vi "Configure Signal (Common).vi"(0 "niUsrpRio Session":T3={"FPGA Interface"=refnum, "RIO Interface Number"=0, "Data Clock Rate"=0, "FPGA Data Clock Rate"=0, "Global Settings Register Bus"=refnum, "Radio 0 Settings Register Bus"=refnum, "Radio 1 Settings Register Bus"=refnum, "Radio Settings Bus Semaphore"=refnum, "DB Queues"=[], "Characterization Data Valid?"=FALSE, "EEPROM Header"={"Checksum"=0, "Product Code"=0, "Hardware Current Version"=0, "Hardware Oldest Compatible Version"=0, "EEPROM Map Current Version"=0, "EEPROM Map Oldest Compatible Version"=0, "User Password"="", "Pointer to Factory Header"=0, "Pointer to User Header"=0, "Recommended Interval"=0, "Number of Reserved Bytes"=9, "Number of Daughterboards"=0, "Daughterboard IDs"=[], "Daughterboard Serial Numbers"=[]}, "Device Data Header"={"Checksum"=0, "Number of Channels"=0, "Number of Gain Settings"=[], "Pointer to Characterization Data"=[], "Number of Reserved Bytes"=27, "Number of Frequencies"=[]}, "EEPROM Characterization Header"={"Checksum"=0, "Date"=timestamp(0 s since 1904-01-01), "Temperature"=0.0, "Misc. Info"="", "Pointer to Device Data Header"=0, "Number of Reserved Bytes"=28}, "Characterization Data"=[], "FPGA Current Version"=0, "FPGA Oldest Compatible Version"=0, "Fixed Logic Current Version"=0, "Fixed Logic Oldest Compatible Version"=0, "FPGA Radio Settings Bus Current Version"=0, "FPGA Radio Settings Bus Oldest Compatible Version"=0, "FPGA Board Config Current Version"=0, "FPGA Board Config Oldest Compatible Version"=0, "Daughterboard Clock Rate"=0, "daughterboard configuration session handles"=[]} {"Daughterboard Clock Rate" format="%#.3pHz"; "FPGA Data Clock Rate" format="%#.3pHz"; "Data Clock Rate" format="%#.3pHz"; "Characterization Data"."Frequencies [Hz]" format="%#_6p"; "EEPROM Characterization Header"."Pointer to Device Data Header" format="%x"; "EEPROM Characterization Header"."Checksum" format="%x"; "Device Data Header"."Pointer to Characterization Data" format="%x"; "Device Data Header"."Checksum" format="%x"; "EEPROM Header"."Pointer to User Header" format="%x"; "EEPROM Header"."Pointer to Factory Header" format="%x"; "EEPROM Header"."Product Code" format="%x"; "EEPROM Header"."Checksum" format="%x"}, 1 "scope":string(combo)="rx", 2 "Correct Impairments?":bool=TRUE, 5 "signal parameters":T2={"gain/level"=0.0, "sample rate [S/s]"=10000000.0, "frequency [Hz]"=2450000000.0, "LO frequency [Hz]"=-1.0, "active antenna"="RX1"} {"LO frequency [Hz]" format="%#.3pHz"; "frequency [Hz]" format="%#.3pHz"; "sample rate [S/s]" min=1.0 max=250000000.0 format="%#.3pS/s"}, 7 "Configure Signal Mode":T1, 11 "error in":errorcluster) -> (4 "niUsrpRio Session (out)":T3={"FPGA Interface"=refnum, "RIO Interface Number"=0, "Data Clock Rate"=0, "FPGA Data Clock Rate"=0, "Global Settings Register Bus"=refnum, "Radio 0 Settings Register Bus"=refnum, "Radio 1 Settings Register Bus"=refnum, "Radio Settings Bus Semaphore"=refnum, "DB Queues"=[], "Characterization Data Valid?"=FALSE, "EEPROM Header"={"Checksum"=0, "Product Code"=0, "Hardware Current Version"=0, "Hardware Oldest Compatible Version"=0, "EEPROM Map Current Version"=0, "EEPROM Map Oldest Compatible Version"=0, "User Password"="", "Pointer to Factory Header"=0, "Pointer to User Header"=0, "Recommended Interval"=0, "Number of Reserved Bytes"=9, "Number of Daughterboards"=0, "Daughterboard IDs"=[], "Daughterboard Serial Numbers"=[]}, "Device Data Header"={"Checksum"=0, "Number of Channels"=0, "Number of Gain Settings"=[], "Pointer to Characterization Data"=[], "Number of Reserved Bytes"=27, "Number of Frequencies"=[]}, "EEPROM Characterization Header"={"Checksum"=0, "Date"=timestamp(0 s since 1904-01-01), "Temperature"=0.0, "Misc. Info"="", "Pointer to Device Data Header"=0, "Number of Reserved Bytes"=28}, "Characterization Data"=[], "FPGA Current Version"=0, "FPGA Oldest Compatible Version"=0, "Fixed Logic Current Version"=0, "Fixed Logic Oldest Compatible Version"=0, "FPGA Radio Settings Bus Current Version"=0, "FPGA Radio Settings Bus Oldest Compatible Version"=0, "FPGA Board Config Current Version"=0, "FPGA Board Config Oldest Compatible Version"=0, "Daughterboard Clock Rate"=0, "daughterboard configuration session handles"=[]} {"Daughterboard Clock Rate" format="%#.3pHz"; "FPGA Data Clock Rate" format="%#.3pHz"; "Data Clock Rate" format="%#.3pHz"; "Characterization Data"."Frequencies [Hz]" format="%#_6p"; "EEPROM Characterization Header"."Pointer to Device Data Header" format="%x"; "EEPROM Characterization Header"."Checksum" format="%x"; "Device Data Header"."Pointer to Characterization Data" format="%x"; "Device Data Header"."Checksum" format="%x"; "EEPROM Header"."Pointer to User Header" format="%x"; "EEPROM Header"."Pointer to Factory Header" format="%x"; "EEPROM Header"."Product Code" format="%x"; "EEPROM Header"."Checksum" format="%x"}, 6 "coerced signal parameters":T2={"gain/level"=0.0, "sample rate [S/s]"=10000000.0, "frequency [Hz]"=2450000000.0, "LO frequency [Hz]"=-1.0, "active antenna"="RX1"} {"LO frequency [Hz]" format="%#.3pHz"; "frequency [Hz]" format="%#.3pHz"; "sample rate [S/s]" min=1.0 max=250000000.0 format="%#.3pS/s"}, 15 "error out":errorcluster)   [LabVIEW 2021]
doc: "Configures the DSP and signal path for the channel based on the input <B>signal parameters</B>.\n\n<B>Input Parameters</B>\n\n<B>Sample Rate</B> the requested rate, in samples per second, the signal will be sampled at.\n\n<B>Frequency</B> is the requested frequency, in hertz, to acquire the signal from/generate the signal at.\n\n<B>Level</B> is the requested power level, in dBm, of the signal.\n\n<B>Gain</B> is the requested amount of gain, in dB.\n\n<B>LO Frequency</B> is the requested frequency, in hertz, to tune the local oscillator to. The default value of -1 sets the LO to the value of the 'Frequency' input. If the value is not -1, the LO will be set to that value, and the DSP will handle the difference between the 'Frequency' and the 'LO Frequency'.\n\n<B>Active Antenna</B> is the antenna to use for this channel.\n\n<B>Correct Impairments</B> applies the correction information of the device to the signal."
uses:
  <instrlib>/niUsrpRio/Config/v1/Host/Public/niUsrpRio Session.ctl
  <instrlib>/_niInstr/Register Bus/v0/Host/Public/Register Bus Session.ctl
  <instrlib>/_niInstr/Register Bus/v0/Host/Private/Session Data.ctl
  <instrlib>/niUsrpRio/Config/v1/Host/Private/DB Queue Reference.ctl
  <instrlib>/niUsrpRio/Config/v1/Host/Private/Daughterboard Data.ctl
  <instrlib>/niUsrpRio/Config/v1/Host/Private/ATR state data.ctl
  <instrlib>/niUsrpRio/Config/v1/Host/Private/Antenna Configuration.ctl
  <instrlib>/niUsrpRio/Config/v1/Host/Private/CPLD Power Mode.ctl
  <instrlib>/niUsrpRio/Config/v1/Host/Public/EEPROM Header.ctl
  <instrlib>/niUsrpRio/Config/v1/Host/Public/EEPROM Device Data Header.ctl
  <instrlib>/niUsrpRio/Config/v1/Host/Public/EEPROM Characterization Header.ctl
  <instrlib>/niUsrpRio/Config/v1/Host/Public/Characterization Data.ctl
  <instrlib>/niUsrpRio/Config/v1/Host/Public/IQ Imbalance.ctl
  Configure Signal Parameters.ctl
  Configure Signal Mode.ctl
  Streaming Xvcr FPGA Ref.ctl
  <instrlib>/_niInstr/DSP/v1/Shared/Public/IQ Impairments.ctl
  <instrlib>/_niInstr/DSP/v1/Shared/Public/IQ Gain.ctl
  <vilib>/Utility/error.llb/Error Cluster From Error Code.vi
  <vilib>/rvi/errors/niLvFpgaAdjustHostInterfaceError.vi
  <vilib>/rvi/interface/nirviReadWriteControl/nirviReadWriteControl.xnode
  <vilib>/ErrorRing/Error Ring.xnode
  NiFpgaLv.dll
  <vilib>/rvi/interface/Simulation/niFpgaSimulationCallBeginRW.vi
  <instrlib>/_niInstr/DSP/v1/Shared/niInstr DSP v1 Shared.lvlib
  <instrlib>/niUsrpRio/Config/v1/Host/niUsrpRio Config v1 Host.lvlib
  <instrlib>/_niInstr/Register Bus/v0/Host/niInstr Register Bus v0 Host.lvlib
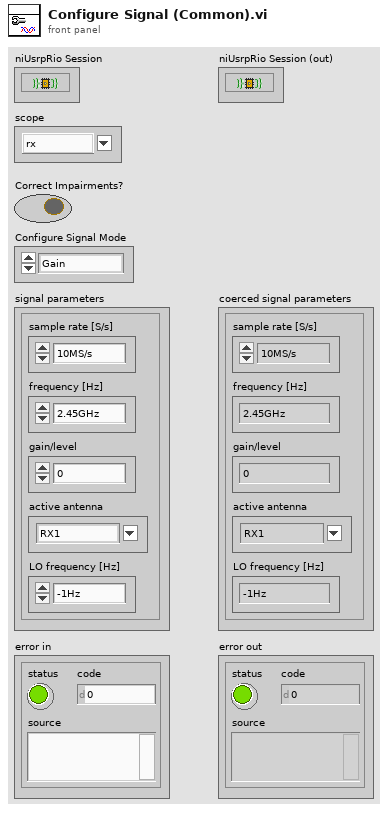
[diagram p1: front panel]
types:
  T1 = typedef "Configure Signal Mode.ctl" = enum16{"Gain", "Level"}
  T2 = typedef "Configure Signal Parameters.ctl" = cluster{"gain/level":dbl, "sample rate [S/s]":dbl, "frequency [Hz]":dbl, "LO frequency [Hz]":dbl, "active antenna":string}
  T3 = typedef "niUsrpRio Config v1 Host.lvlib/niUsrpRio Session.ctl" = cluster{"FPGA Interface":refnum<k20>, "RIO Interface Number":u32, "Data Clock Rate":u32, "FPGA Data Clock Rate":u32, "Global Settings Register Bus":T4, "Radio 0 Settings Register Bus":T4, "Radio 1 Settings Register Bus":T4, "Radio Settings Bus Semaphore":T5, "DB Queues":T6[], "Characterization Data Valid?":bool, "EEPROM Header":T7, "Device Data Header":T8, "EEPROM Characterization Header":T9, "Characterization Data":T10[], "FPGA Current Version":u32, "FPGA Oldest Compatible Version":u32, "Fixed Logic Current Version":u32, "Fixed Logic Oldest Compatible Version":u32, "FPGA Radio Settings Bus Current Version":u32, "FPGA Radio Settings Bus Oldest Compatible Version":u32, "FPGA Board Config Current Version":u32, "FPGA Board Config Oldest Compatible Version":u32, "Daughterboard Clock Rate":u32, "daughterboard configuration session handles":u64[]}
  T4 = typedef "niInstr Register Bus v0 Host.lvlib/Register Bus Session.ctl" = refnum<queue>
  T5 = typedef "Semaphore RefNum" = refnum<k1>
  T6 = typedef "niUsrpRio Config v1 Host.lvlib/DB Queue Reference.ctl" = refnum<queue>
  T7 = typedef "niUsrpRio Config v1 Host.lvlib/EEPROM Header.ctl" = cluster{"Checksum":u32, "Product Code":u16, "Hardware Current Version":u16, "Hardware Oldest Compatible Version":u16, "EEPROM Map Current Version":u16, "EEPROM Map Oldest Compatible Version":u16, "User Password":string, "Pointer to Factory Header":u32, "Pointer to User Header":u32, "Recommended Interval":u16, "Number of Reserved Bytes":i32, "Number of Daughterboards":u8, "Daughterboard IDs":u16[], "Daughterboard Serial Numbers":string[]}
  T8 = typedef "niUsrpRio Config v1 Host.lvlib/EEPROM Device Data Header.ctl" = cluster{"Checksum":u32, "Number of Channels":u8, "Number of Gain Settings":u16[], "Pointer to Characterization Data":u32[], "Number of Reserved Bytes":i32, "Number of Frequencies":u16[]}
  T9 = typedef "niUsrpRio Config v1 Host.lvlib/EEPROM Characterization Header.ctl" = cluster{"Checksum":u32, "Date":timestamp, "Temperature":sgl, "Misc. Info":string, "Pointer to Device Data Header":u32, "Number of Reserved Bytes":i32}
  T10 = typedef "niUsrpRio Config v1 Host.lvlib/Characterization Data.ctl" = cluster{"Gains[dB]":dbl[], "Frequencies [Hz]":dbl[], "IQ Imbalance Table":T11[], "Measured Gains[dB]":dbl[][]}
  T11 = typedef "niUsrpRio Config v1 Host.lvlib/IQ Imbalance.ctl" = cluster{"Gain Imbalance [linear]":dbl, "Phase Imbalance [radians]":dbl, "Offset":cdb}
  T12 = typedef "Streaming Xvcr FPGA Ref.ctl" = refnum<k20>
  T13 = typedef "niInstr DSP v1 Shared.lvlib/IQ Impairments.ctl" = cluster{"inline gain I":fxp<+/-,18,1>, "inline gain Q":fxp<+/-,18,1>, "cross gain I":fxp<+/-,18,1>, "cross gain Q":fxp<+/-,18,1>, "pre-gain offset I":fxp<+/-,18,1>, "pre-gain offset Q":fxp<+/-,18,1>, "post-gain offset I":fxp<+/-,18,1>, "post-gain offset Q":fxp<+/-,18,1>}
  T14 = typedef "niUsrpRio Config v1 Host.lvlib/DB Types.ctl" = enum16{"sbx", "cbx", "wbx", "unknown", "ubx", "twinrx"}
  T15 = typedef "niUsrpRio Config v1 Host.lvlib/Device Subfunction.ctl" = enum16{"rx", "tx", "all"}
  T16 = typedef "niUsrpRio Config v1 Host.lvlib/RF Channel 2.ctl" = enum16{"0", "1", "2", "3", "All"}
  T17 = typedef "niInstr DSP v1 Shared.lvlib/IQ Gain.ctl" = cluster{"gain I":fxp<+/-,24,3>, "gain Q":fxp<+/-,24,3>}
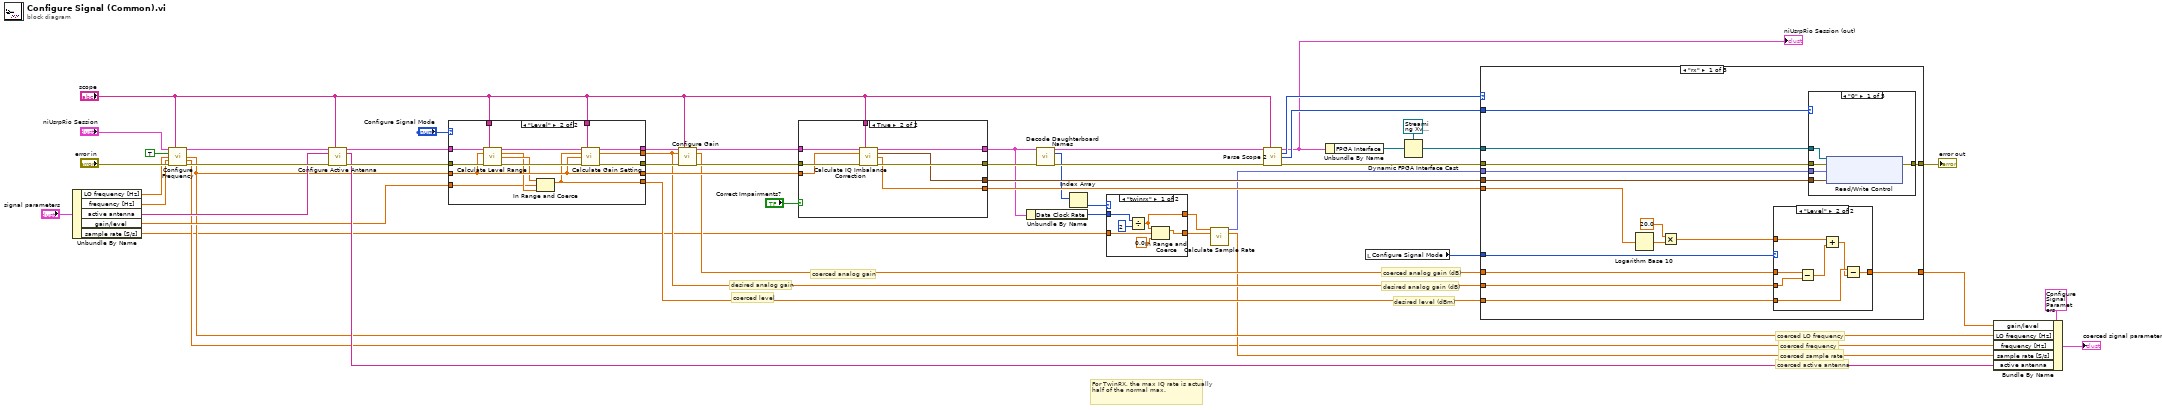
[diagram p0: block diagram]
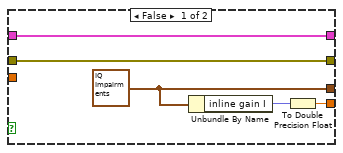
[diagram p3: hidden frame]
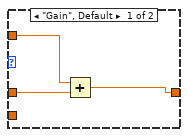
[diagram p5: hidden frame]
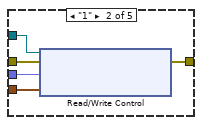
[diagram p6: hidden frame]
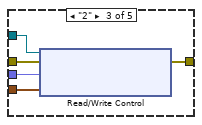
[diagram p7: hidden frame]
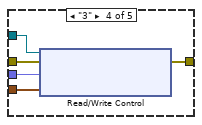
[diagram p8: hidden frame]
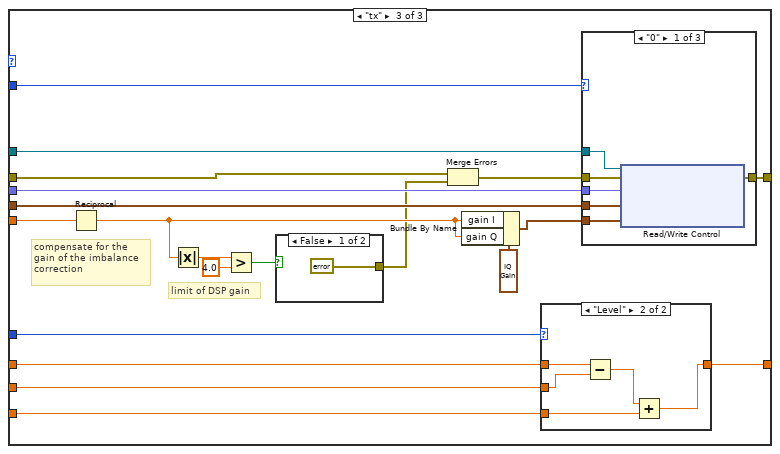
[diagram p11: hidden frame]
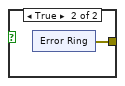
[diagram p12: hidden frame]
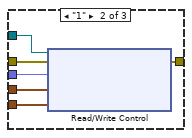
[diagram p14: hidden frame]
diagram:
  # "For TwinRX, the max IQ rate is actually half of the normal max."
  # "coerced level"
  # "desired level (dBm)"
  # "desired analog gain"
  # "desired analog gain (dB)"
  # "coerced analog gain (dB)"
  # "coerced analog gain"
  # "coerced active antenna"
  # "coerced sample rate"
  # "coerced frequency"
  # "coerced LO frequency"
  n1 = Unbundle By Name("signal parameters") -> ("LO frequency [Hz]"=w39:dbl, "frequency [Hz]"=w28:dbl, "active antenna"=w38:string, "gain/level"=w22:dbl, "sample rate [S/s]"=w6:dbl)
  n2 = call "Configure Frequency.vi"("niUsrpRio Session"="niUsrpRio Session", "scope"="scope", "wait for lo to lock"=TRUE, "lo frequency"=w39, "frequency"=w28, "error in"="error in") -> ("niUsrpRio Session (out)"=w45:T3, "coerced lo frequency"=w20:dbl, "coerced frequency"=w11:dbl, "error out"=w44:errorcluster)  [unwired: 6 in]
  n3 = call <instrlib>:"Configure Active Antenna.vi"("niUsrpRio Session"=w45, "scope"="scope", "active antenna"=w38, "error in"=w44) -> ("niUsrpRio Session (out)"=w36:T3, "coerced active antenna"=w27:string, "error out"=w35:errorcluster)  [unwired: 9 in]
  n4 = case shown="\"Level\"" "Configure Signal Mode" {
    tunnel: w36 -> [w55 w60]
    tunnel: w35 -> [w54 w69]
    tunnel: w22 -> [w53 w61]
    tunnel: "scope" -> [_ w66]
    tunnel: [w55 w65] -> w32
    tunnel: w20 -> [w56 w67]
    tunnel: [w56 w67] -> w34
    tunnel: [w54 w70] -> w33
    tunnel: [w53 w64] -> w23
    tunnel: "scope" -> [_ w58]
    tunnel: [w53 w57] -> w17
    frame "Gain", Default {
    }
    frame "Level" {
      n5 = call <instrlib>:"Calculate Level Range.vi"("niUsrpRio Session"=w60, "scope"=w58, "frequency"=w67, "error in"=w69) -> ("niUsrpRio Session (out)"=w59:T3, "Min Level"=w62:dbl, "Max Level"=w63:dbl, "error out"=w68:errorcluster)  [unwired: 8 in]
      n6 = In Range and Coerce(upper limit=w63, x=w61, lower limit=w62) -> (coerced(x)=w57:dbl)  [unwired: 1 out]
      n7 = call <instrlib>:"Calculate Gain Setting.vi"("niUsrpRio Session"=w59, "scope"=w66, "level"=w57, "frequency"=w67, "error in"=w68) -> ("niUsrpRio Session (out)"=w65:T3, "gain"=w64:dbl, "error out"=w70:errorcluster)  [unwired: 8 in]
    }
  }
  n8 = call <instrlib>:"Configure Gain.vi"("niUsrpRio Session"=w32, "scope"="scope", "gain"=w23, "error in"=w33) -> ("niUsrpRio Session (out)"=w31:T3, "coerced gain"=w24:dbl, "error out"=w30:errorcluster)  [unwired: 9 in]
  n9 = case shown="True" "Correct Impairments?" {
    tunnel: w30 -> [w74 w82]
    tunnel: w31 -> [w75 w83]
    tunnel: "scope" -> [_ w81]
    tunnel: [w75 w80] -> w1
    tunnel: [w74 w79] -> w10
    tunnel: [w71 w78] -> w42
    tunnel: [w72 w76] -> w41
    tunnel: w34 -> [_ w77]
    frame False {
      w71 = T13 {"inline gain I"=0.9999923706054688, "inline gain Q"=0.9999923706054688, "cross gain I"=0.0, "cross gain Q"=0.0, "pre-gain offset I"=0.0, "pre-gain offset Q"=0.0, "post-gain offset I"=0.0, "post-gain offset Q"=0.0} ("impairment control")
      n10 = Unbundle By Name(w71) -> ("inline gain I"=w73:fxp<+/-,18,1>)
      n11 = To Double Precision Float(number=w73) -> (double precision float=w72:dbl)
    }
    frame True {
      n12 = call <instrlib>:"Calculate IQ Imbalance Correction.vi"("niUsrpRio Session"=w83, "scope"=w81, "frequency"=w77, "error in"=w82) -> ("niUsrpRio Session (out)"=w80:T3, "IQ imbalance correction"=w78:T13, "correction gain"=w76:dbl, "error out"=w79:errorcluster)  [unwired: 8 in]
    }
  }
  n13 = Unbundle By Name(w1) -> ("Data Clock Rate"=w4:u32)
  n14 = call <instrlib>:"Decode Daughterboard Names.vi"("niUsrpRio Session"=w1, "error in"=w10) -> ("niUsrpRio Session (out)"=w2:T3, "daughterboard names"=w8:T14[], "error out"=w9:errorcluster)  [unwired: 10 in, 1 out]
  n15 = Index Array(array=w8) -> (element=w5:T14)  [unwired: 1 in]
  n16 = case shown="\"twinrx\"" w5 {
    tunnel: [w88 w91] -> w7
    tunnel: w6 -> [w89 w91]
    tunnel: w4 -> [w86 w90]
    tunnel: [w84 w90] -> w3
    frame "twinrx" {
      n17 = Divide(x=w86, y=u32 2) -> (x/y=w84:dbl)
      n18 = In Range and Coerce(upper limit=w84, x=w89, lower limit=0.0) -> (coerced(x)=w88:dbl)  [unwired: 1 out]
    }
    frame Default {
    }
  }
  n19 = call "Calculate Sample Rate.vi"("data clock rate"=w3, "sample rate"=w7) -> ("decimation sample rate"=w12:fxp<+,48,1>, "coerced sample rate"=w13:dbl)  [unwired: 12 in]
  n20 = call <instrlib>:"Parse Scope 2.vi"("niUsrpRio Session"=w2, "scope"="scope", "error in"=w9) -> ("niUsrpRio Session (out)"=w47:T3, "Device Subfunction"=w49:T15, "Device Subfunction Channel"=w48:T16, "error out"=w46:errorcluster)  [unwired: 4 in, 5 out]
  "niUsrpRio Session (out)" <- w47
  n21 = Unbundle By Name(w47) -> ("FPGA Interface"=w16:refnum<k20>)
  n22 = local read "Configure Signal Mode"() -> (w25:T1)
  n23 = Dynamic FPGA Interface Cast(Session In=T12 refnum ("FPGA VI Reference Out"), Type=w16) -> (Session Out=w15:T12)
  n24 = case shown="\"rx\"" w49 {
    tunnel: w12 -> [w106 _ w158]
    tunnel: w15 -> [w105 _ w139]
    tunnel: [w104 w138 w157] -> w52
    tunnel: w46 -> [w103 w138 w156]
    tunnel: w42 -> [w102 _ w155]
    tunnel: w48 -> [w101 _ w154]
    tunnel: w41 -> [w95 _ w152]
    tunnel: w25 -> [w99 _ w150]
    tunnel: w24 -> [w100 _ w149]
    tunnel: [w98 _ w148] -> w21
    tunnel: w23 -> [w96 _ w147]
    tunnel: w17 -> [w97 _ w146]
    frame "rx" {
      n25 = Logarithm Base 10(1:w95) -> (0:w93:dbl)
      n26 = Multiply(x=20.0, y=w93) -> (x*y=w92:dbl)
      n27 = case shown="\"Level\"" w99 {
        tunnel: w100 -> [w108 w116]
        tunnel: [w107 w110] -> w98
        tunnel: w96 -> [_ w115]
        tunnel: w97 -> [_ w112]
        tunnel: w92 -> [w109 w114]
        frame "Gain", Default {
          n28 = Add(x=w109, y=w108) -> (x+y=w107:dbl)
        }
        frame "Level" {
          n29 = Subtract(x=w116, y=w115) -> (x-y=w113:dbl)
          n30 = Add(x=w114, y=w113) -> (x+y=w111:dbl)
          n31 = Subtract(x=w112, y=w111) -> (x-y=w110:dbl)
        }
      }
      n32 = case shown="\"0\"" w101 {
        tunnel: w106 -> [w119 w126 w131 w136 _]
        tunnel: [w117 w125 w130 w135 w137] -> w104
        tunnel: w103 -> [w121 w124 w129 w134 w137]
        tunnel: w105 -> [w120 w123 w128 w133 _]
        tunnel: w102 -> [w118 w122 w127 w132 _]
        frame "0" {
          n33 = xnode "Read/Write Control"("FPGA VI Reference In"=w120, "error in"=w121, "rx.output sample rate"=w119, "rx 0.impairments"=w118) -> ("error out"=w117:errorcluster)  [unwired: 1 out]
        }
        frame "1" {
          n34 = xnode "Read/Write Control"("FPGA VI Reference In"=w123, "error in"=w124, "rx.output sample rate"=w126, "rx 1.impairments"=w122) -> ("error out"=w125:errorcluster)  [unwired: 1 out]
        }
        frame "2" {
          n35 = xnode "Read/Write Control"("FPGA VI Reference In"=w128, "error in"=w129, "rx.output sample rate"=w131, "rx 2.impairments"=w127) -> ("error out"=w130:errorcluster)  [unwired: 1 out]
        }
        frame "3" {
          n36 = xnode "Read/Write Control"("FPGA VI Reference In"=w133, "error in"=w134, "rx.output sample rate"=w136, "rx 3.impairments"=w132) -> ("error out"=w135:errorcluster)  [unwired: 1 out]
        }
        frame Default {
        }
      }
    }
    frame Default {
    }
    frame "tx" {
      # "limit of DSP gain"
      # "compensate for the\ngain of the imbalance\ncorrection"
      n37 = Reciprocal(x=w152) -> (1/x=w144:dbl)
      n38 = Absolute Value(x=w144) -> (abs(x)=w142:dbl)
      n39 = Greater?(x=w142, y=4.0) -> (0:w145:bool)
      n40 = case shown="False" w145 {
        tunnel: [errorcluster {"status"=FALSE, "code"=0, "source"=""} ("error constant") w160] -> w140
        frame False {
        }
        frame True {
          n41 = xnode "Error Ring"() -> ("error out"=w160:errorcluster)
        }
      }
      n42 = Merge Errors(w156, w140) -> (w141:errorcluster)
      n43 = Bundle By Name(cluster=T17 {"gain I"=1.0, "gain Q"=1.0} ("gain"), "gain I"=w144, "gain Q"=w144) -> (w151:T17)
      n44 = case shown="\"Level\"" w150 {
        tunnel: w149 -> [w166 w171]
        tunnel: [w166 w167] -> w148
        tunnel: w147 -> [_ w170]
        tunnel: w146 -> [_ w169]
        frame "Gain", Default {
        }
        frame "Level" {
          n45 = Subtract(x=w171, y=w170) -> (x-y=w168:dbl)
          n46 = Add(x=w168, y=w169) -> (x+y=w167:dbl)
        }
      }
      n47 = case shown="\"0\"" w154 {
        tunnel: w158 -> [w177 w183 _]
        tunnel: [w176 w182 w184] -> w157
        tunnel: w141 -> [w175 w181 w184]
        tunnel: w139 -> [w174 w180 _]
        tunnel: w155 -> [w173 w179 _]
        tunnel: w151 -> [w172 w178 _]
        frame "0" {
          n48 = xnode "Read/Write Control"("FPGA VI Reference In"=w174, "error in"=w175, "tx.input sample rate"=w177, "tx 0.impairments"=w173, "tx 0.gain"=w172) -> ("error out"=w176:errorcluster)  [unwired: 1 out]
        }
        frame "1" {
          n49 = xnode "Read/Write Control"("FPGA VI Reference In"=w180, "error in"=w181, "tx.input sample rate"=w183, "tx 1.impairments"=w179, "tx 1.gain"=w178) -> ("error out"=w182:errorcluster)  [unwired: 1 out]
        }
        frame Default {
        }
      }
    }
  }
  "error out" <- w52
  n50 = Bundle By Name(cluster=T2 {"gain/level"=0.0, "sample rate [S/s]"=10000000.0, "frequency [Hz]"=2450000000.0, "LO frequency [Hz]"=-1.0, "active antenna"="RX1"} ("coerced signal parameters"), "gain/level"=w21, "LO frequency [Hz]"=w20, "frequency [Hz]"=w11, "sample rate [S/s]"=w13, "active antenna"=w27) -> (→"coerced signal parameters":T2)
